vi "Stop DC_1_Brake.vi"(2 "DC Motor":cluster{"DC Motor":T2, "Address":i16}={"DC Motor"=enum."DC Motor", "Address"=-1}, 3 "NXT":T1={"Hardware"="NXT", "Flattened String"=""}) -> (0 "NXT":T1={"Hardware"="NXT", "Flattened String"=""})   [LabVIEW 2010, in "4134Outputs.lvlib"]
uses:
  <vilib>/NXT/Subs/MotorXNode.DC Motor Type.ctl
  <vilib>/NXT/Subs/LVHSConnector.ctl
  4134Outputs.lvlib
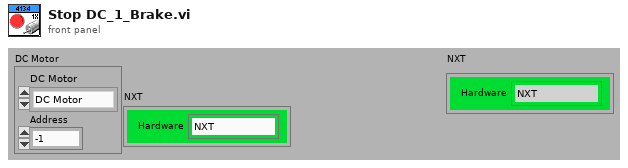
[diagram p1: front panel]
types:
  T1 = typedef "LVHSConnector.ctl" = cluster{"Hardware":string, "Flattened String":string}
  T2 = typedef "MotorXNode.DC Motor Type.ctl" = enum16{"DC Motor"}
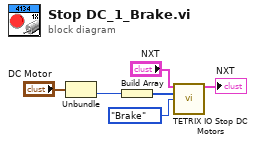
[diagram p0: block diagram]
diagram:
  n1 = Unbundle("DC Motor") -> ("Address"=w5:i16)  [unwired: 1 out]
  n2 = Build Array(w5) -> (w3:i16[])
  n3 = call <vilib>:"TETRIX IO Stop DC Motors.vi"("NXT"="NXT", "DC Motors"=w3, "Stopping Style"=enum16{"Coast", "Brake"}."Brake") -> ("NXT"=→"NXT":T1)  [unwired: 12 in]
